vi "1.1-Act.vi"() -> ()   [LabVIEW 2010]
uses:
  <vilib>/addons/control/pid/fpga.llb/XNode/niFpgaPID.xnode
  <vilib>/eio/EIONode/EIONode.xnode
  <vilib>/rvi/eio/nirviEIOImplementation/nirviEIOImplementation.xnode
  <vilib>/rvi/eio/common/nirviEmuClasses.ctl
  1.0-Hindbrain Global.vi
  <vilib>/rvi/eio/common/nirviEmuTemplateMethod_noerrors.vi
panel:
  in  "Drive gains":T1={"proportional gain (Kc)"=1.0, "integral gain (Kc*Ts/Ti)"=1.66796875, "derivative gain (Kc*Td/Ts)"=0.0} {"proportional gain (Kc)" format="%.11g"; "integral gain (Kc*Ts/Ti)" format="%.11g"; "derivative gain (Kc*Td/Ts)" format="%.11g"}
  in  "Steering gains":T1={"proportional gain (Kc)"=1.0, "integral gain (Kc*Ts/Ti)"=1.66796875, "derivative gain (Kc*Td/Ts)"=0.0} {"proportional gain (Kc)" format="%.11g"; "integral gain (Kc*Ts/Ti)" format="%.11g"; "derivative gain (Kc*Td/Ts)" format="%.11g"}
  # "e"
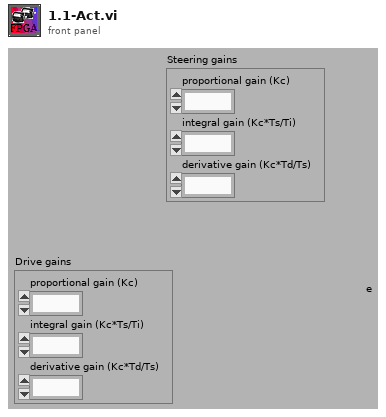
[diagram p1: front panel]
types:
  T1 = cluster{"proportional gain (Kc)":fxp<+/-,16,8>, "integral gain (Kc*Ts/Ti)":fxp<+/-,16,8>, "derivative gain (Kc*Td/Ts)":fxp<+/-,16,8>}
  T2 = typedef "nirviEmuClasses.ctl" = enum16{"IO Read", "IO Write", "Method", "Property Read", "Property Write"}
  T3 = cluster{"proportional gain (Kc)":i16, "integral gain (Kc*Ts/Ti)":i16, "derivative gain (Kc*Td/Ts)":i16}
  T4 = typedef "2.4-How Sensor Typedef.ctl" = cluster{"Motor Speed Integer":i16, "Drive Position Integer":i32, "Lidar Position Integer":i32, "Steering Position Integer":i32, "Battery Voltage Fxp":fxp<+/-,16,5>, "Drive Control Voltage":fxp<+/-,20,5>, "Steering Control Voltage":fxp<+/-,20,5>, "Drive Encoder Cable Check":bool, "Lidar Drive Encoder Cable Check":bool, "Steer Encoder Cable Check":bool, "Lidar Pos Encoder Cable Check":bool, "Mod Buttons & Blinky Cable Check":bool, "Lidar Data Cable Check":bool, "Drive Motor Cable Check":bool, "Vector Nav Cable Check":bool, "Lidar Drive Cable Check":bool, "Steer Drive Cable Check":bool}
  T5 = typedef "2.1-Act Command Typedef.ctl" = cluster{"Steering Integer Setpoint":i16, "Drive Speed Integer Setpoint":i16, "Lidar Position Integer Setpoint":i16, "Inhibit All Motors":bool, "Drive Direct":fxp<+/-,20,5>, "Steer Direct":fxp<+/-,20,5>, "Lidar Direct ":fxp<+/-,20,5>, "2.1 Voltage Pass Through (Joystick)":bool}
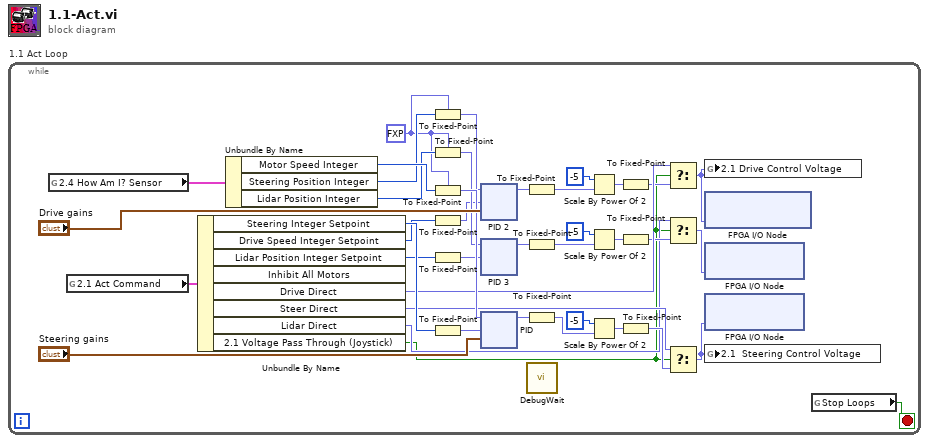
[diagram p0: block diagram]
diagram:
  n1 = while "1.1 Act Loop" {
    stop <- w40 stop-if-true
    w26 = fxp<+/-,16,16> 0.0 ("process variable")
    n2 = global read "1.0-Hindbrain Global.vi" "2.4 How Am I? Sensor"() -> (w38:T4)
    n3 = global read "1.0-Hindbrain Global.vi" "2.1 Act Command"() -> (w39:T5)
    n4 = Unbundle By Name(w39) -> ("Steering Integer Setpoint"=w34:i16, "Drive Speed Integer Setpoint"=w33:i16, "Lidar Position Integer Setpoint"=w32:i16, "Drive Direct"=w16:fxp<+/-,20,5>, "Steer Direct"=w10:fxp<+/-,20,5>, "Lidar Direct"=w2:fxp<+/-,20,5>, "2.1 Voltage Pass Through (Joystick)"=w1:bool)  [unwired: 1 out]
    n5 = Unbundle By Name(w38) -> ("Motor Speed Integer"=w35:i16, "Steering Position Integer"=w30:i32, "Lidar Position Integer"=w29:i32)
    n6 = To Fixed-Point(fixed-point type=w26, number=w30) -> (fixed-point=w25:fxp<+/-,16,16>)
    n7 = To Fixed-Point(fixed-point type=w26, number=w29) -> (fixed-point=w28:fxp<+/-,16,16>)
    n8 = To Fixed-Point(fixed-point type=w26, number=w35) -> (fixed-point=w31:fxp<+/-,16,16>)
    n9 = To Fixed-Point(number=w33) -> (fixed-point=w17:fxp<+/-,16,16>)  [unwired: 1 in]
    n10 = To Fixed-Point(number=w32) -> (fixed-point=w27:fxp<+/-,16,16>)  [unwired: 1 in]
    n11 = To Fixed-Point(number=w34) -> (fixed-point=w18:fxp<+/-,16,16>)  [unwired: 1 in]
    n12 = xnode ("PID 2")("process variable"=w25, "setpoint"=w17, "PID gains"="Drive gains") -> ("output"=w15:fxp<+/-,16,16>)  [unwired: 2 in]
    n13 = xnode ("PID 3")("process variable"=w28, "setpoint"=w27) -> ("output"=w5:fxp<+/-,16,16>)  [unwired: 3 in]
    n14 = xnode ("PID")("process variable"=w31, "setpoint"=w18, "PID gains"="Steering gains") -> ("output"=w12:fxp<+/-,16,16>)  [unwired: 2 in]
    n15 = To Fixed-Point(number=w15) -> (fixed-point=w24:fxp<+/-,21,16>)  [unwired: 1 in]
    n16 = To Fixed-Point(number=w5) -> (fixed-point=w6:fxp<+/-,21,16>)  [unwired: 1 in]
    n17 = To Fixed-Point(number=w12) -> (fixed-point=w19:fxp<+/-,21,16>)  [unwired: 1 in]
    n18 = call "DebugWait.vi"() -> ()  [unwired: 12 in]
    n19 = Scale By Power Of 2(n=-5, x=w24) -> (x*2^n=w22:fxp<+/-,21,16>)
    n20 = Scale By Power Of 2(n=-5, x=w6) -> (x*2^n=w8:fxp<+/-,21,16>)
    n21 = Scale By Power Of 2(n=-5, x=w19) -> (x*2^n=w21:fxp<+/-,21,16>)
    n22 = To Fixed-Point(number=w22) -> (fixed-point=w14:fxp<+/-,20,5>)  [unwired: 1 in]
    n23 = To Fixed-Point(number=w8) -> (fixed-point=w4:fxp<+/-,20,5>)  [unwired: 1 in]
    n24 = To Fixed-Point(number=w21) -> (fixed-point=w11:fxp<+/-,20,5>)  [unwired: 1 in]
    n25 = Select(t=w16, s=w1, f=w14) -> (s? t:f=w13:fxp<+/-,20,5>)
    n26 = Select(t=w2, s=w1, f=w4) -> (s? t:f=w3:fxp<+/-,20,5>)
    n27 = Select(t=w10, s=w1, f=w11) -> (s? t:f=w9:fxp<+/-,20,5>)
    n28 = global write "1.0-Hindbrain Global.vi" "2.1 Drive Control Voltage"(w13) -> ()
    n29 = xnode "FPGA I/O Node"("Drive Motor"=w13) -> ()  [unwired: 1 in, 1 out]
    n30 = xnode "FPGA I/O Node"("Lidar Drive"=w3) -> ()  [unwired: 1 in, 1 out]
    n31 = xnode "FPGA I/O Node"("Steer Drive"=w9) -> ()  [unwired: 1 in, 1 out]
    n32 = global write "1.0-Hindbrain Global.vi" "2.1  Steering Control Voltage"(w9) -> ()
    n33 = global read "1.0-Hindbrain Global.vi" "Stop Loops"() -> (w40:bool)
  }
